vi "Read Step Data(DC Program).vi"(5 "Step Number":u32=1 min=1 max=24, 7 "Mem Number":u32=1 min=1 max=50, 8 "Error In":errorcluster, 11 "VISA resource name":refnum<visa-resource-name>) -> (0 "Error Out":errorcluster, 2 "AC Advance Step Data":T1 {"Transient Time" format="%.1f ms"; "Transient Site" format="%.0f ¢X"; "Transient Volt" format="%.1f V"; "CF Lo Limit" format="%.2f"; "CF Hi Limit" format="%.2f"; "Q Lo Limit" format="%.0f VAR"; "Q Hi Limit" format="%.0f VAR"; "VA Lo Limit" format="%.0f VA"; "VA Hi Limit" format="%.0f VA"; "PF Lo Limit" format="%.3f"; "PF Hi Limit" format="%.3f"; "P Lo Limit" format="%.0f W"; "P Hi Limit" format="%.0f W"; "AP Lo Limit" format="%.1f A"; "AP Hi Limit" format="%.1f A"; "A Lo Limit" format="%.2f A"; "A Hi Limit" format="%.2f A"; "Delay Time" format="%.1f s"; "£GT" format="%.0f ms"; "£GF" format="%.1f Hz"; "£GV" format="%.1f V"; "Time" format="%.1f s"; "Voltage" format="%.1f V"; "Frequency" format="%.1f Hz"}, 3 "VISA resource name out":refnum<visa-resource-name>)   [LabVIEW 2013]
uses:
  Utility/Get Step Address(DC Program).vi
panel:
  in  "Modbus ID":string
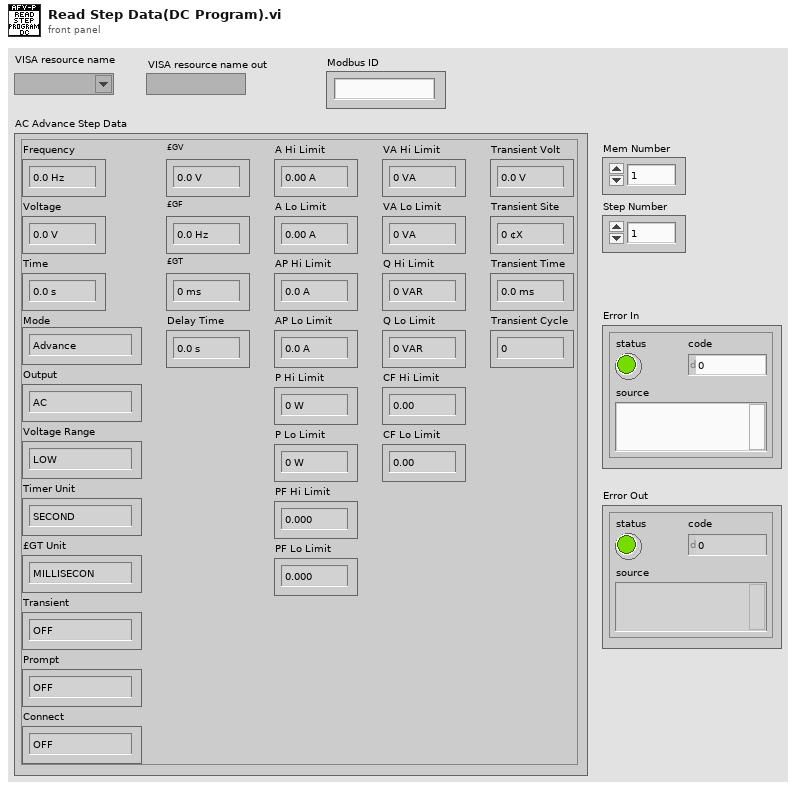
[diagram p1: front panel]
types:
  T1 = cluster{"Frequency":dbl, "Voltage":dbl, "Time":dbl, "Mode":enum16{"Advance", "Basic"}, "Output":enum16{"AC", "DC"}, "Voltage Range":enum16{"LOW", "HIGH", "AUTO"}, "Timer Unit":enum16{"SECOND", "MINUTE", "HOUR"}, "£GT Unit":enum16{"MILLISECON", "SECOND", "CYCLE"}, "Transient":enum16{"OFF", "ON"}, "Prompt":enum16{"OFF", "ON"}, "Connect":enum16{"OFF", "ON"}, "£GV":dbl, "£GF":dbl, "£GT":u16, "Delay Time":dbl, "A Hi Limit":dbl, "A Lo Limit":dbl, "AP Hi Limit":dbl, "AP Lo Limit":dbl, "P Hi Limit":u16, "P Lo Limit":u16, "PF Hi Limit":dbl, "PF Lo Limit":dbl, "VA Hi Limit":u16, "VA Lo Limit":u16, "Q Hi Limit":u16, "Q Lo Limit":u16, "CF Hi Limit":dbl, "CF Lo Limit":dbl, "Transient Volt":dbl, "Transient Site":u16, "Transient Time":dbl, "Transient Cycle":u16}
  T2 = cluster{"ID":string, "Function Code":string, "Length (High)":string, "Length (Low)":string, "Start Address (High)":string, "Start Address (Middle High)":string, "Start Address (Middle Low)":string, "Start Address (Low)":string, "Data":string}
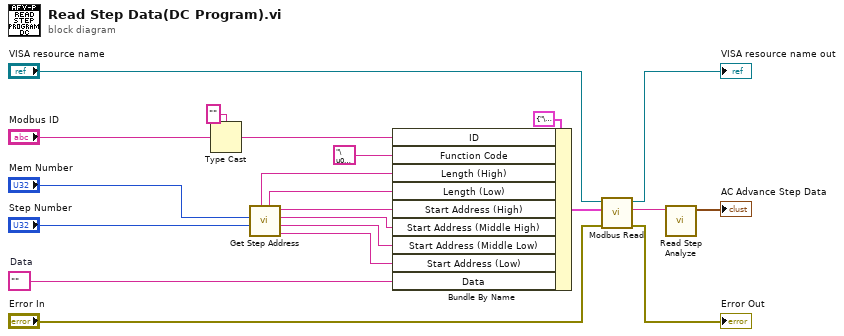
[diagram p0: block diagram]
diagram:
  w21 = ""  # Data
  n1 = Type Cast(type="" ("Binary Data (Hex) 3"), x="Modbus ID") -> (*(type *) &x=w9:string)
  n2 = call-poly "Get Step Address.vi"("Program Data.Step Number"="Step Number", "Program Data.Mem Number"="Mem Number") -> ("Program Data.Start Address (Low)"=w3:string, "Program Data.Start Address (Middle Low)"=w2:string, "Program Data.Start Address (Middle High)"=w1:string, "Program Data.Start Address (High)"=w4:string, "Length (Low)"=w5:string, "Length (High)"=w6:string)  [unwired: 4 in]
  n3 = Bundle By Name(cluster=T2 {"ID"="\u0000", "Function Code"="\u0000", "Length (High)"="\u0000", "Length (Low)"="\u0000", "Start Address (High)"="\u0000", "Start Address (Middle High)"="\u0000", "Start Address (Middle Low)"="\u0000", "Start Address (Low)"="\u0000", "Data"=""} ("Write Buffer"), "ID"=w9, "Function Code"="\u0003", "Length (High)"=w6, "Length (Low)"=w5, "Start Address (High)"=w4, "Start Address (Middle High)"=w1, "Start Address (Middle Low)"=w2, "Start Address (Low)"=w3, "Data"=w21) -> (w18:T2)
  n4 = call "Modbus Read.vi"("Error In"="Error In", "Write Buffer"=w18, "VISA resource name"="VISA resource name") -> ("Error Out"=→"Error Out":errorcluster, "Read Data"=w13:string, "VISA resource name out"=→"VISA resource name out":refnum<visa-resource-name>)  [unwired: 6 in]
  n5 = call "Read Step Analyze.vi"("Data"=w13) -> ("AC Advance Step Data"=→"AC Advance Step Data":T1)  [unwired: 10 in]
